vi "Compare Auto-Index and Last Value.vi"() -> ()   [LabVIEW 2019]
panel:
  out "Output Tunnel Result (Last Value)":i32
  out "Input Tunnel Result (No Auto Index)":dbl[](array[numeric])
  out "Output Tunnel Result":i32[](array[numeric])
  in  "1D DBL Array Input":dbl[](array[numeric])=[25.0, 50.0, 75.0, 100.0, 125.0, 150.0, 175.0, 200.0, 225.0, 250.0, 275.0, 300.0]
  out "Input Tunnel Result (Auto Index)":dbl
  out "Current Iteration":i32
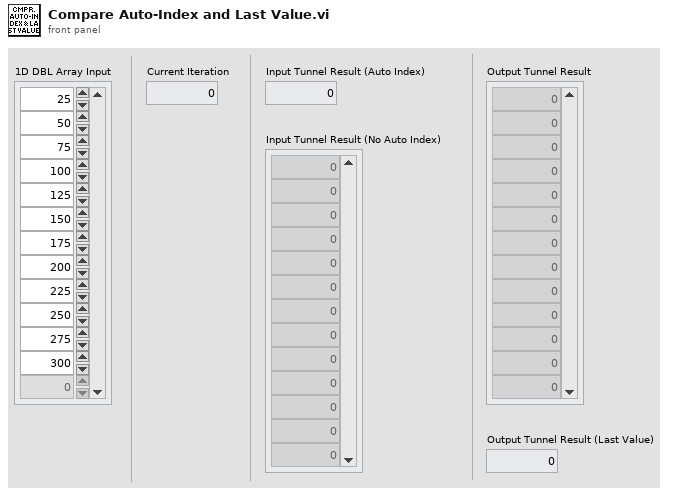
[diagram p1: front panel]
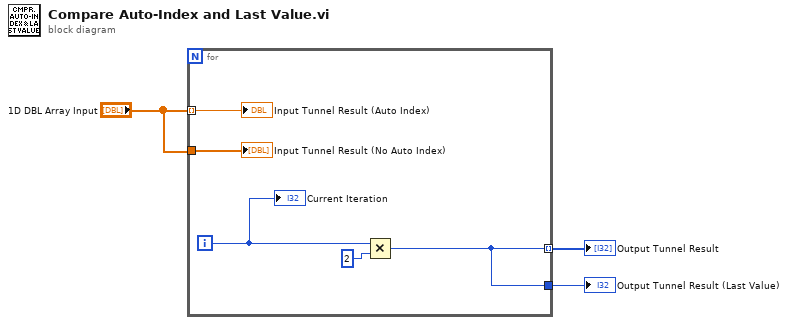
[diagram p0: block diagram]
diagram:
  n1 = for {
    tunnel: "1D DBL Array Input" -> [w6] mode=indexing
    tunnel: [w4] -> w3 mode=indexing
    tunnel: "1D DBL Array Input" -> [w5]
    tunnel: [w4] -> w1
    i -> [w8]
    n2 = Multiply(x=w8, y=2) -> (x*y=w4:i32)
    "Input Tunnel Result (Auto Index)" <- w6
    "Current Iteration" <- w8
    "Input Tunnel Result (No Auto Index)" <- w5
  }
  "Output Tunnel Result" <- w3
  "Output Tunnel Result (Last Value)" <- w1
